vi "LAN Config TCPIP.vi"(0 "VISA resource name":refnum<visa-resource-name>, 1 "IP Address":string="10.1.1.10", 2 "Subnet Mask":string="255.255.255.0", 3 "Default Gateway":string="10.1.1.1", 5 "Node In":string, 7 "Config Method (Automatic)":enum16{"Automatic", "Manual"}(ring), 11 "error in":errorcluster, 12 "DNS Address 1":string="10.1.1.2", 13 "DNS Address 2":string="10.1.1.3") -> (4 "VISA resource name out":refnum<visa-resource-name>, 6 "Node Out":string, 14 "Command String":string, 15 "error out":errorcluster)   [LabVIEW 2012, in "Keithley 2600 Series.lvlib"]
doc: "This VI configures the instrument's TCP/IP settings.\n\n<b>Note:</b> You will need to call LAN Apply Settings for these settings to take effect.\n\n<b>Functions and Attributes Used</b>\nlan.config.method\nlan.config.ipaddress\nlan.config.gateway\nlan.config.subnetmask\nlan.config.dns.address[N]"
uses:
  Keithley 2600 Series.lvlib
  Private/GlobalVariables.vi
panel:
  # "(c) 2008 Keithley Instruments, Inc.  ALL RIGHTS RESERVED."
  # "Manual Settings"
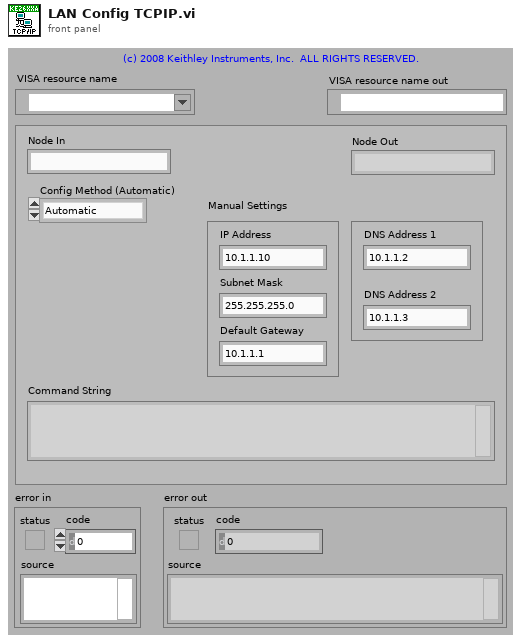
[diagram p1: front panel]
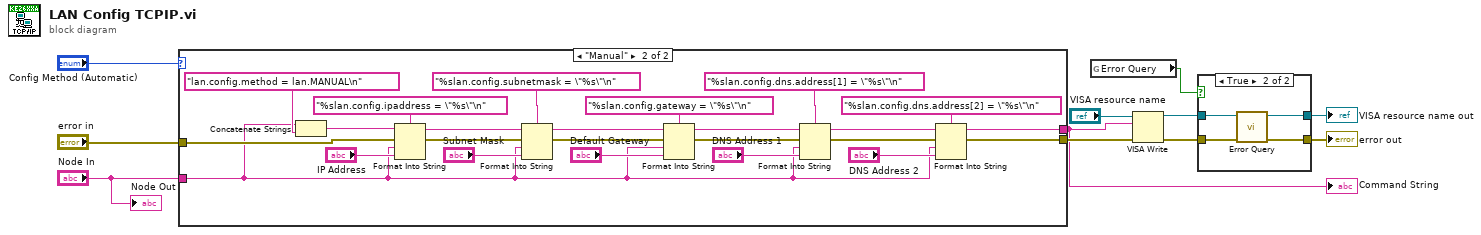
[diagram p0: block diagram]
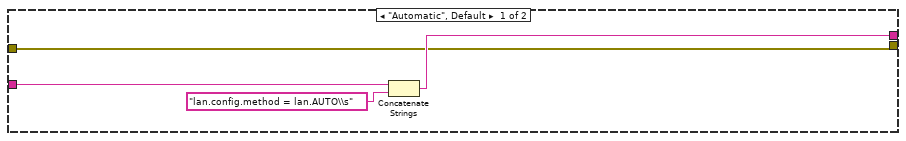
[diagram p3: hidden frame]
diagram:
  n1 = case shown="\"Manual\"" "Config Method (Automatic)" {
    tunnel: "Node In" -> [w15 w18]
    tunnel: [w13 w17] -> w1
    tunnel: "error in" -> [w12 w23]
    tunnel: [w12 w16] -> w8
    frame "Automatic", Default {
      n2 = Concatenate Strings(w15, "lan.config.method = lan.AUTO\\s") -> (w13:string)
    }
    frame "Manual" {
      n3 = Concatenate Strings(w18, "lan.config.method = lan.MANUAL\n") -> (w28:string)
      n4 = Format Into String(format string="%slan.config.ipaddress = \"%s\"\n", initial string=w28, error in=w23, w18, "IP Address") -> (resulting string=w27:string, error out=w22:errorcluster)
      n5 = Format Into String(format string="%slan.config.subnetmask = \"%s\"\n", initial string=w27, error in=w22, w18, "Subnet Mask") -> (resulting string=w26:string, error out=w21:errorcluster)
      n6 = Format Into String(format string="%slan.config.gateway = \"%s\"\n", initial string=w26, error in=w21, w18, "Default Gateway") -> (resulting string=w25:string, error out=w20:errorcluster)
      n7 = Format Into String(format string="%slan.config.dns.address[1] = \"%s\"\n", initial string=w25, error in=w20, w18, "DNS Address 1") -> (resulting string=w24:string, error out=w19:errorcluster)
      n8 = Format Into String(format string="%slan.config.dns.address[2] = \"%s\"\n", initial string=w24, error in=w19, w18, "DNS Address 2") -> (resulting string=w17:string, error out=w16:errorcluster)
    }
  }
  "Command String" <- w1
  n9 = global read "GlobalVariables.vi" "Error Query"() -> (w6:bool)
  n10 = VISA Write(VISA resource name="VISA resource name", write buffer=w1, error in (no error)=w8) -> (VISA resource name out=w5:refnum<visa-resource-name>, error out=w4:errorcluster)  [unwired: 1 out]
  n11 = case shown="True" w6 {
    tunnel: w5 -> [w41 w45]
    tunnel: w4 -> [w40 w44]
    tunnel: [w41 w43] -> w3
    tunnel: [w40 w42] -> w2
    frame False {
    }
    frame True {
      n12 = call "Error Query.vi"("error in (no error)"=w44, "VISA resource name"=w45) -> ("error out"=w42:errorcluster, "VISA resource name out"=w43:refnum<visa-resource-name>)  [unwired: 8 out]
    }
  }
  "VISA resource name out" <- w3
  "error out" <- w2
  "Node Out" <- "Node In"
